vi "PLC_Status.vi"(1 "appended array":refnum<vi>[](array[refnum]), 5 "Machine name":string[](array[string]), 7 "Station number":string[](array[string]), 9 "IP Address":string[](array[string]), 11 "error in (no error)":errorcluster, 12 "PLC Status":errorcluster[](array[cluster]), 14 "Recipe Names":string[][](array[string])) -> (15 "error out":errorcluster)   [LabVIEW 2017]
panel:
  in  "PLC":bool
  in  "PRODUCT LIST":string(combo)
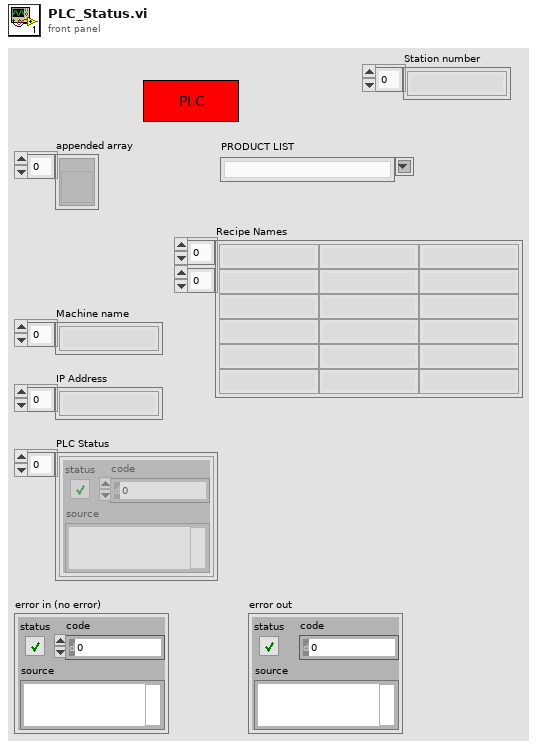
[diagram p1: front panel]
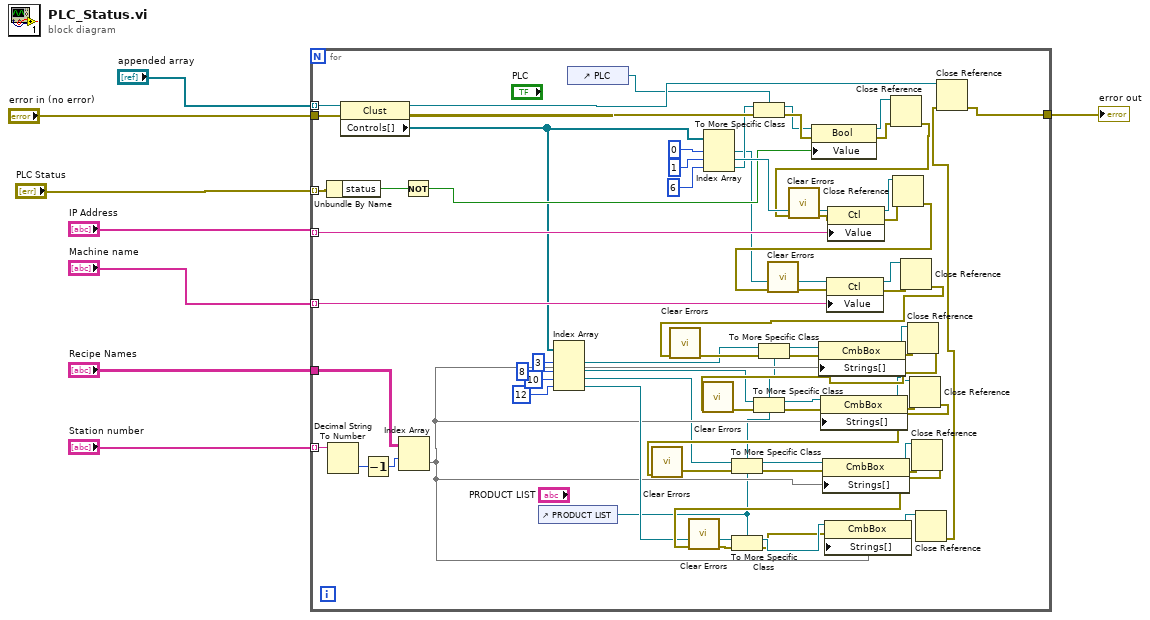
[diagram p0: block diagram]
diagram:
  n1 = for {
    tunnel: [w67] -> w6
    tunnel: "appended array" -> [w76] mode=indexing
    tunnel: "error in (no error)" -> [w74]
    tunnel: "PLC Status" -> [w70] mode=indexing
    tunnel: "IP Address" -> [w63] mode=indexing
    tunnel: "Machine name" -> [w57] mode=indexing
    tunnel: "Recipe Names" -> [w29]
    tunnel: "Station number" -> [w33] mode=indexing
    n2 = Unbundle By Name(w70) -> ("status"=w69:bool)
    n3 = Decimal String To Number(string=w33) -> (number=w35:i32)  [unwired: 2 in, 1 out]
    n4 = property class="Clust"(reference=w76, error in=w74) -> (reference out=w66:refnum<vi>, error out=w73:errorcluster, "Controls[]"=w46:refnum<vi>[])
    n5 = Decrement(x=w35) -> (x-1=w34:i32)
    n6 = Index Array(array=w29, index (row)=w34) -> (element=w25:string[])  [unwired: 1 in]
    n7 = Not(x=w69) -> (.not. x?=w56:bool)
    n8 = control-ref of="PRODUCT LIST"() -> (w10:refnum<vi>)
    n9 = Index Array(array=w46, index #1=3 ("index"), index #2=8 ("index"), index #3=10 ("index"), index #4=12 ("index")) -> (element #1=w11:refnum<vi>, element #2=w15:refnum<vi>, element #3=w20:refnum<vi>, element #4=w28:refnum<vi>)
    n10 = control-ref of="PLC"() -> (w9:refnum<vi>)
    n11 = Index Array(array=w46, index #1=0 ("index"), index #2=1 ("index"), index #3=6 ("index")) -> (element #1=w49:refnum<vi>, element #2=w64:refnum<vi>, element #3=w50:refnum<vi>)
    n12 = To More Specific Class(target class=w9, reference=w50, error in=w73) -> (specific class reference=w71:refnum<vi>, error out=w72:errorcluster)
    n13 = property class="Bool"(reference=w71, error in=w72, "Value"=w56) -> (reference out=w68:refnum<vi>, error out=w55:errorcluster)
    n14 = Close Reference(reference=w68, error in (no error)=w55) -> (error out=w53:errorcluster)
    n15 = call <vilib>:"Clear Errors.vi"("error in (no error)"=w53) -> ("error out"=w54:errorcluster)  [unwired: 5 in, 1 out]
    n16 = property class="Ctl"(reference=w64, error in=w54, "Value"=w63) -> (reference out=w61:refnum<vi>, error out=w62:errorcluster)
    n17 = Close Reference(reference=w61, error in (no error)=w62) -> (error out=w52:errorcluster)
    n18 = call <vilib>:"Clear Errors.vi"("error in (no error)"=w52) -> ("error out"=w51:errorcluster)  [unwired: 5 in, 1 out]
    n19 = property class="Ctl"(reference=w49, error in=w51, "Value"=w57) -> (reference out=w60:refnum<vi>, error out=w59:errorcluster)
    n20 = Close Reference(reference=w60, error in (no error)=w59) -> (error out=w47:errorcluster)
    n21 = call <vilib>:"Clear Errors.vi"("error in (no error)"=w47) -> ("error out"=w14:errorcluster)  [unwired: 5 in, 1 out]
    n22 = To More Specific Class(target class=w10, reference=w11, error in=w14) -> (specific class reference=w12:refnum<vi>, error out=w13:errorcluster)
    n23 = property class="CmbBox"(reference=w12, error in=w13, "Strings[]"=w25) -> (reference out=w32:refnum<vi>, error out=w48:errorcluster)
    n24 = Close Reference(reference=w32, error in (no error)=w48) -> (error out=w38:errorcluster)
    n25 = call <vilib>:"Clear Errors.vi"("error in (no error)"=w38) -> ("error out"=w18:errorcluster)  [unwired: 5 in, 1 out]
    n26 = To More Specific Class(target class=w10, reference=w15, error in=w18) -> (specific class reference=w16:refnum<vi>, error out=w17:errorcluster)
    n27 = property class="CmbBox"(reference=w16, error in=w17, "Strings[]"=w25) -> (reference out=w31:refnum<vi>, error out=w41:errorcluster)
    n28 = Close Reference(reference=w31, error in (no error)=w41) -> (error out=w37:errorcluster)
    n29 = call <vilib>:"Clear Errors.vi"("error in (no error)"=w37) -> ("error out"=w21:errorcluster)  [unwired: 5 in, 1 out]
    n30 = To More Specific Class(target class=w10, reference=w20, error in=w21) -> (specific class reference=w19:refnum<vi>, error out=w22:errorcluster)
    n31 = property class="CmbBox"(reference=w19, error in=w22, "Strings[]"=w25) -> (reference out=w30:refnum<vi>, error out=w40:errorcluster)
    n32 = Close Reference(reference=w30, error in (no error)=w40) -> (error out=w36:errorcluster)
    n33 = call <vilib>:"Clear Errors.vi"("error in (no error)"=w36) -> ("error out"=w24:errorcluster)  [unwired: 5 in, 1 out]
    n34 = To More Specific Class(target class=w10, reference=w28, error in=w24) -> (specific class reference=w26:refnum<vi>, error out=w23:errorcluster)
    n35 = property on="Property Node" class="CmbBox"(reference=w26, error in=w23, "Strings[]"=w25) -> (reference out=w27:refnum<vi>)  [unwired: 1 out]
    n36 = Close Reference(reference=w27) -> (error out=w39:errorcluster)  [unwired: 1 in]
    n37 = Close Reference(reference=w66, error in (no error)=w39) -> (error out=w67:errorcluster)
  }
  "error out" <- w6
